vi "HOTEL.vi"() -> ()   [LabVIEW 2020]
panel:
  in  "?":dbl
  out "?":string
  out "?":dbl
  in  "?":dbl
  out "?":string
  out "?":dbl
  in  "?":dbl
  out "?":string
  out "?":dbl
  in  "?":dbl
  out "?":string
  out "?":dbl
  in  "?":dbl
  out "?":string
  out "?":dbl
  in  "?":dbl
  out "?":string
  out "?":dbl
  in  "?":dbl
  out "?":string
  out "?":dbl
  in  "?":dbl
  out "?":string
  out "?":dbl
  out "TOTAL CALORIES":dbl
  out "TOTAL AMOUNT":dbl
  in  "?":bool
  in  "?":dbl
  out "?":string
  out "?":dbl
  out "?":dbl
  out "?":string
  in  "?":dbl
  # "BREAKFAST"
  # "ITEMS"
  # "ITEM PRICE"
  # "QUANTITY"
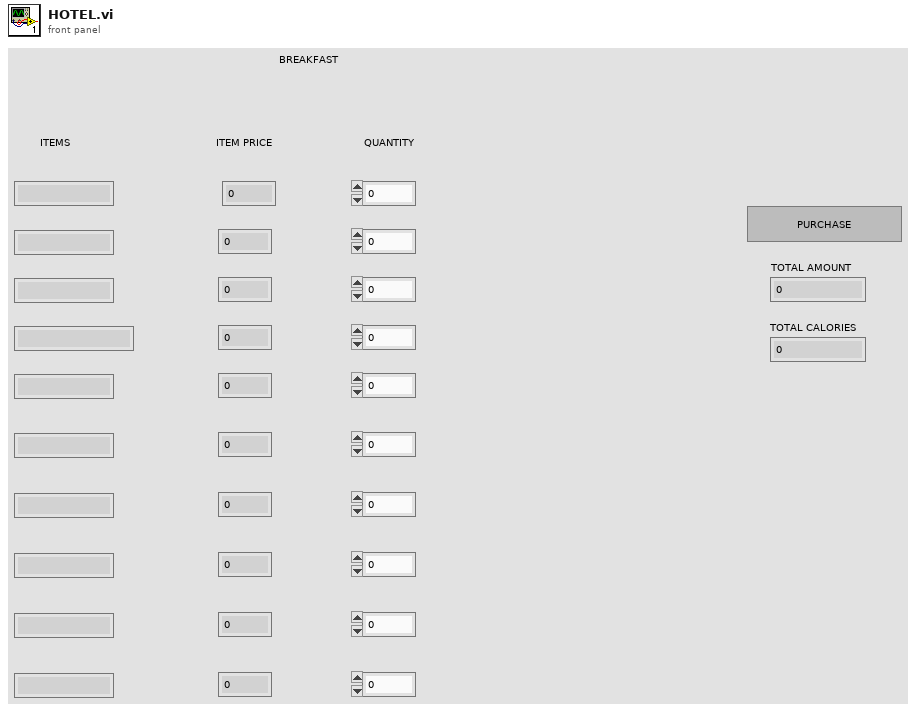
[diagram p1: front panel]
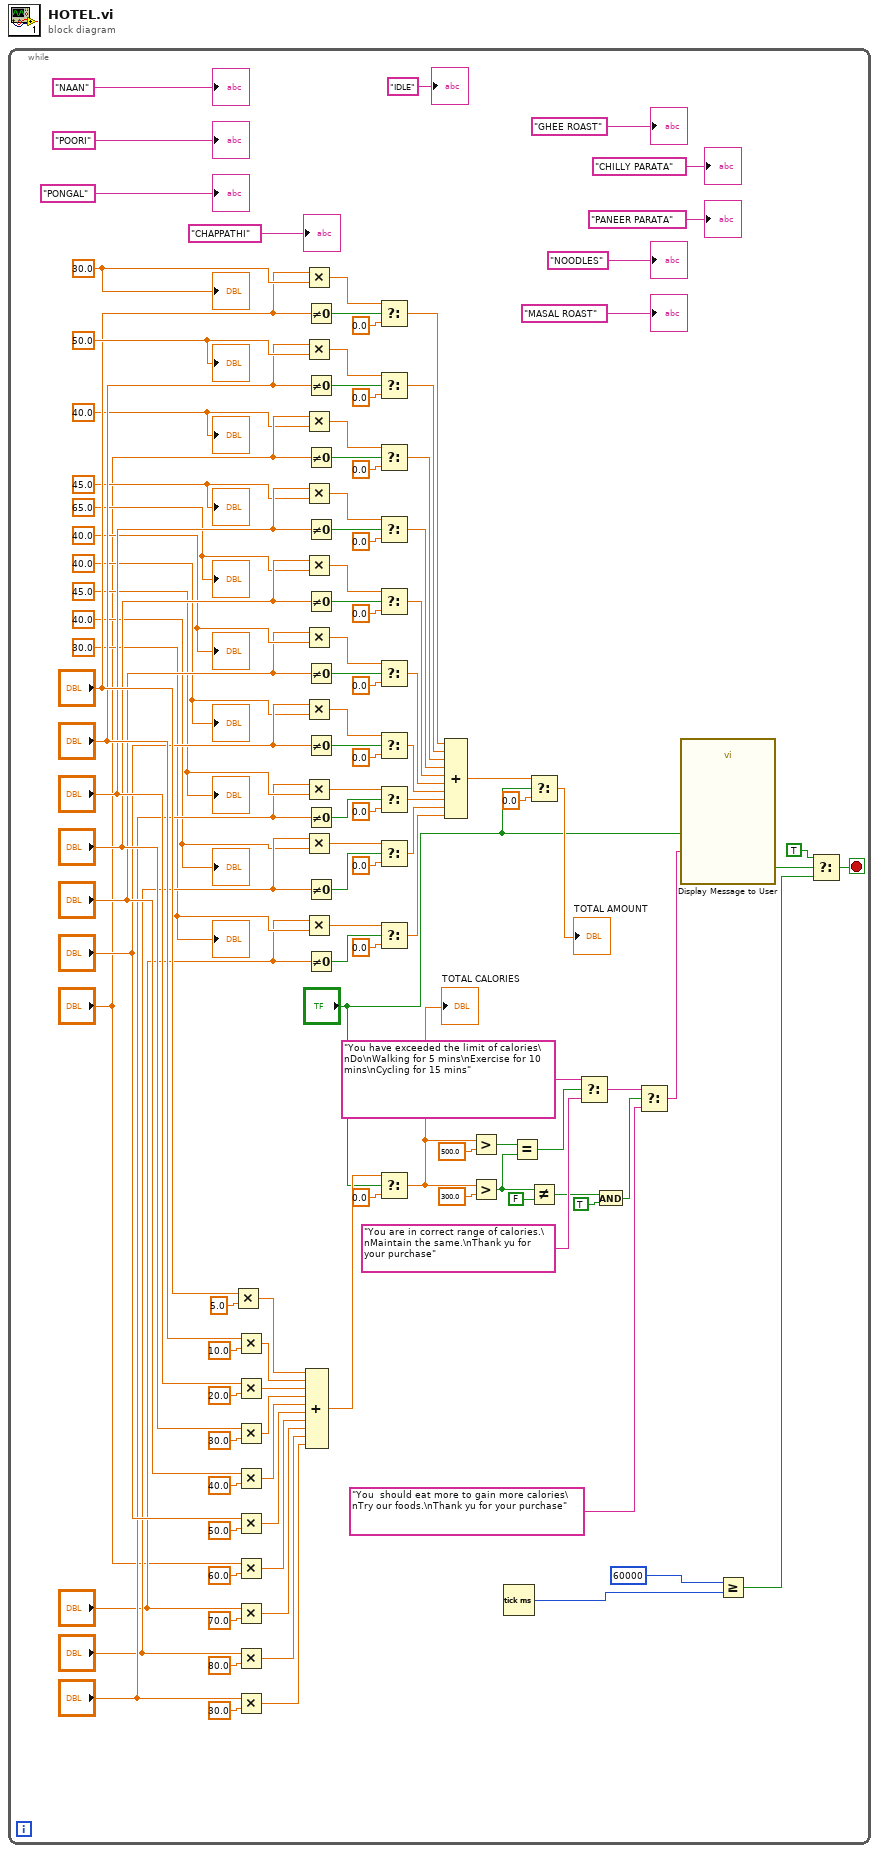
[diagram p0: block diagram]
diagram:
  n1 = while {
    stop <- w7 stop-if-true
    w44 = 40.0
    w56 = 30.0
    w57 = 40.0
    w70 = 45.0
    w71 = 40.0
    w83 = 40.0
    w84 = 65.0
    w92 = 45.0
    w111 = 50.0
    w116 = 30.0
    n2 = Multiply(x="?", y=5.0) -> (x*y=w103:dbl)
    n3 = Multiply(x="?", y=10.0) -> (x*y=w102:dbl)
    n4 = Multiply(x="?", y=20.0) -> (x*y=w43:dbl)
    n5 = Multiply(x="?", y=30.0) -> (x*y=w42:dbl)
    n6 = Multiply(x="?", y=40.0) -> (x*y=w41:dbl)
    n7 = Multiply(x="?", y=50.0) -> (x*y=w40:dbl)
    n8 = Multiply(x="?", y=60.0) -> (x*y=w39:dbl)
    n9 = Multiply(x="?", y=70.0) -> (x*y=w38:dbl)
    n10 = Multiply(x="?", y=80.0) -> (x*y=w37:dbl)
    n11 = Multiply(x="?", y=30.0) -> (x*y=w36:dbl)
    n12 = Multiply(x="?", y=w116) -> (x*y=w115:dbl)
    n13 = Multiply(x="?", y=w111) -> (x*y=w112:dbl)
    n14 = Multiply(x="?", y=w44) -> (x*y=w46:dbl)
    n15 = Multiply(x="?", y=w92) -> (x*y=w91:dbl)
    n16 = Multiply(x="?", y=w84) -> (x*y=w88:dbl)
    n17 = Multiply(x="?", y=w83) -> (x*y=w79:dbl)
    n18 = Multiply(x="?", y=w71) -> (x*y=w73:dbl)
    n19 = Multiply(x="?", y=w70) -> (x*y=w68:dbl)
    n20 = Multiply(x="?", y=w57) -> (x*y=w59:dbl)
    n21 = Multiply(x="?", y=w56) -> (x*y=w54:dbl)
    n22 = Not Equal To 0?(x="?") -> (x != 0?=w117:bool)
    n23 = Not Equal To 0?(x="?") -> (x != 0?=w110:bool)
    n24 = Not Equal To 0?(x="?") -> (x != 0?=w47:bool)
    n25 = Not Equal To 0?(x="?") -> (x != 0?=w93:bool)
    n26 = Not Equal To 0?(x="?") -> (x != 0?=w87:bool)
    n27 = Not Equal To 0?(x="?") -> (x != 0?=w80:bool)
    n28 = Not Equal To 0?(x="?") -> (x != 0?=w74:bool)
    n29 = Not Equal To 0?(x="?") -> (x != 0?=w67:bool)
    n30 = Not Equal To 0?(x="?") -> (x != 0?=w60:bool)
    n31 = Not Equal To 0?(x="?") -> (x != 0?=w53:bool)
    n32 = Compound Arithmetic op=ADD(w103, w102, w43, w42, w41, w40, w39, w38, w37, w36) -> (w97:dbl)
    n33 = Select(t=w115, s=w117, f=0.0) -> (s? t:f=w109:dbl)
    n34 = Select(t=w112, s=w110, f=0.0) -> (s? t:f=w108:dbl)
    n35 = Select(t=w46, s=w47, f=0.0) -> (s? t:f=w35:dbl)
    n36 = Select(t=w91, s=w93, f=0.0) -> (s? t:f=w34:dbl)
    n37 = Select(t=w88, s=w87, f=0.0) -> (s? t:f=w33:dbl)
    n38 = Select(t=w79, s=w80, f=0.0) -> (s? t:f=w32:dbl)
    n39 = Select(t=w73, s=w74, f=0.0) -> (s? t:f=w31:dbl)
    n40 = Select(t=w68, s=w67, f=0.0) -> (s? t:f=w30:dbl)
    n41 = Select(t=w59, s=w60, f=0.0) -> (s? t:f=w29:dbl)
    n42 = Select(t=w54, s=w53, f=0.0) -> (s? t:f=w28:dbl)
    n43 = Select(t=w97, s="?", f=0.0) -> (s? t:f=w26:dbl)
    "TOTAL CALORIES" <- w26
    n44 = Compound Arithmetic op=ADD(w109, w108, w35, w34, w33, w32, w31, w30, w29, w28) -> (w96:dbl)
    n45 = Greater?(x=w26, y=500.0) -> (0:w25:bool)
    n46 = Greater?(x=w26, y=300.0) -> (0:w21:bool)
    n47 = Tick Count (ms)() -> (millisecond timer value=w12:u32)
    n48 = Equal?(x=w25, y=w21) -> (x = y?=w18:bool)
    n49 = Select(t=w96, s="?", f=0.0) -> (s? t:f=→"TOTAL AMOUNT":dbl)
    n50 = Not Equal?(x=w21, y=FALSE) -> (x != y?=w20:bool)
    n51 = Select(t="You have exceeded the limit of calories\nDo\nWalking for 5 mins\nExercise for 10 mins\nCycling for 15 mins", s=w18, f="You are in correct range of calories.\nMaintain the same.\nThank yu for your purchase") -> (s? t:f=w17:string)
    n52 = And(x=w20, y=TRUE) -> (x .and. y?=w19:bool)
    n53 = Select(t=w17, s=w19, f="You  should eat more to gain more calories\nTry our foods.\nThank yu for your purchase") -> (s? t:f=w15:string)
    n54 = call "Display Message to User"("Enable"="?", "Message"=w15) -> ("OK"=w9:bool)  [unwired: 8 in, 1 out]
    n55 = Greater Or Equal?(x=u32 60000 ("milliseconds to wait"), y=w12) -> (x >= y?=w8:bool)
    n56 = Select(t=TRUE, s=w9, f=w8) -> (s? t:f=w7:bool)
    "?" <- w116
    "?" <- w111
    "?" <- w92
    "?" <- w84
    "?" <- w83
    "?" <- "NAAN"
    "?" <- w71
    "?" <- "PONGAL"
    "?" <- w70
    "?" <- "CHAPPATHI"
    "?" <- w57
    "?" <- "POORI"
    "?" <- w56
    "?" <- w44
    "?" <- "IDLE"
    "?" <- "MASAL ROAST"
    "?" <- "PANEER PARATA"
    "?" <- "CHILLY PARATA"
    "?" <- "GHEE ROAST"
    "?" <- "NOODLES"
  }
